vi "RTM CheckCRC.vi"(8 "error in (no error)":errorcluster, 10 "SignalName":string, 11 "Node Ptr":T1 format="%.0x") -> (0 "error out":errorcluster, 2 "CRC?":bool, 3 "Node Ptr 2":T1 format="%.0x")   [LabVIEW 2018, in "CAN Gateway System Explorer.lvlib"]
uses:
  CAN Gateway System Explorer.lvlib
  <vilib>/NI Veristand/Custom Device API/Custom Device Item Ref.ctl
  <vilib>/NI Veristand/Custom Device API/Custom Device API.lvlib
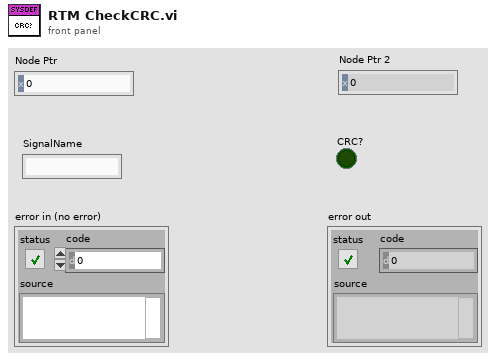
[diagram p1: front panel]
types:
  T1 = typedef "Custom Device API.lvlib/Custom Device Item Ref.ctl" = u64
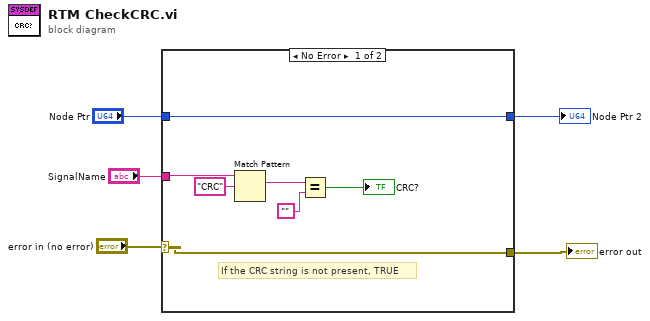
[diagram p0: block diagram]
diagram:
  n1 = case shown="No Error" "error in (no error)" {
    selector: "error in (no error)" -> [w9 w13]
    tunnel: "Node Ptr" -> [w12 w14]
    tunnel: [w12 w14] -> w4
    tunnel: "SignalName" -> [w11 _]
    tunnel: [w9 w13] -> w1
    frame No Error {
      # "If the CRC string is not present, TRUE"
      n2 = Match Pattern(string=w11, regular expression="CRC") -> (match substring=w8:string)  [unwired: 1 in, 3 out]
      n3 = Equal?(x=w8, y="") -> (x = y?=→"CRC?":bool)
    }
    frame Error {
    }
  }
  "error out" <- w1
  "Node Ptr 2" <- w4
